vi "Convert Entry Mode to Cmd.vi"(11 "entry mode":T1(ring)) -> (3 "Numeric":u8)   [LabVIEW 2015, in "HD44780 Common.lvlib"]
uses:
  HD44780 Common.lvlib
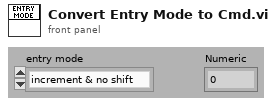
[diagram p1: front panel]
types:
  T1 = enum8{"increment & no shift", "increment & shift", "decrement & no shift", "decrement & shift"}
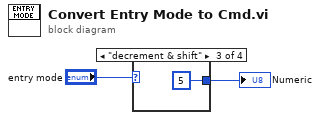
[diagram p0: block diagram]
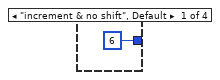
[diagram p2: hidden frame]
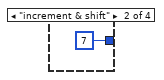
[diagram p3: hidden frame]
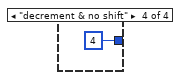
[diagram p4: hidden frame]
diagram:
  n1 = case shown="\"decrement & shift\"" "entry mode" {
    tunnel: [u8 6 u8 7 u8 5 u8 4] -> w2
    frame "increment & no shift", Default {
    }
    frame "increment & shift" {
    }
    frame "decrement & shift" {
    }
    frame "decrement & no shift" {
    }
  }
  "Numeric" <- w2
